vi "Read Horizontal Scrollbar.vi"(11 "Flex Subpanel in":refnum<class "Flex UI Subpanel.lvclass">) -> (2 "Horizontal Scrollbar":bool, 3 "Flex Subpanel out":refnum<class "Flex UI Subpanel.lvclass">)   [LabVIEW 2016, in "Flex UI Subpanel.lvclass"]
uses:
  Flex UI Subpanel.lvclass
  Flex UI Subpanel.lvclass/Flex UI Subpanel.ctl
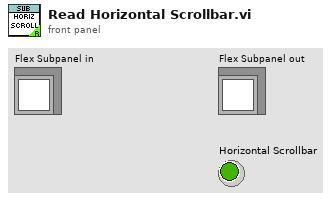
[diagram p1: front panel]
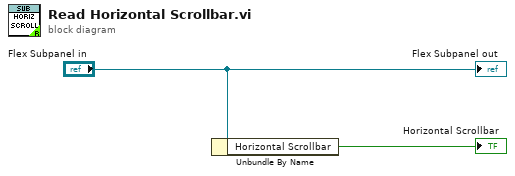
[diagram p0: block diagram]
diagram:
  n1 = Unbundle By Name("Flex Subpanel in") -> ("Horizontal Scrollbar"=→"Horizontal Scrollbar":bool)
  "Flex Subpanel out" <- "Flex Subpanel in"
